vi "Rig - Save or Load.vi"(6 "Saving Rig Config to test directory?":bool, 7 "Rig Settings IN":T1={"Rig Name"="", "Rig Room"="1.4", "Base Directory"="", "Computer IP Address"="", "Globals Name"="", "Treatmill Str"="", "cRIO Test Data Dir"=path "", "ai"="", "ao"="", "dio"="", "A_calib_str_row1"="", "A_calib_str_row2"="0", "A_calib_str_row3"="1.4", "Zero_V_str"="", "step_V"="", "Sample Freq"="", "ai_threshold"="", "run_speed_thresh"="", "speed_time_length"="", "wall ball gain"="", "max wall pos"="", "max cor width"="", "Trial Config Directory"=path "C:/Whisker Tester/Trials", "Randomize Trials?"=FALSE}, 8 "Error IN":errorcluster, 10 "RigSave Path IN":path, 11 "Command IN":T2) -> (0 "Error OUT":errorcluster, 3 "Rig Settings OUT":T1={"Rig Name"="", "Rig Room"="1.4", "Base Directory"="", "Computer IP Address"="", "Globals Name"="", "Treatmill Str"="", "cRIO Test Data Dir"=path "", "ai"="", "ao"="", "dio"="", "A_calib_str_row1"="", "A_calib_str_row2"="0", "A_calib_str_row3"="1.4", "Zero_V_str"="", "step_V"="", "Sample Freq"="", "ai_threshold"="", "run_speed_thresh"="", "speed_time_length"="", "wall ball gain"="", "max wall pos"="", "max cor width"="", "Trial Config Directory"=path "C:/Whisker Tester/Trials", "Randomize Trials?"=FALSE})   [LabVIEW 2018]
uses:
  controls/Command IN_Recipe.ctl
  controls/Rig Config Settings.ctl
  <vilib>/Utility/file.llb/Write Delimited Spreadsheet (string).vi
  <vilib>/Utility/file.llb/Read Delimited Spreadsheet (string).vi
  Globals/Global - Configuration Options.vi
panel:
  # "INPUTS"
  # "OUTPUTS"
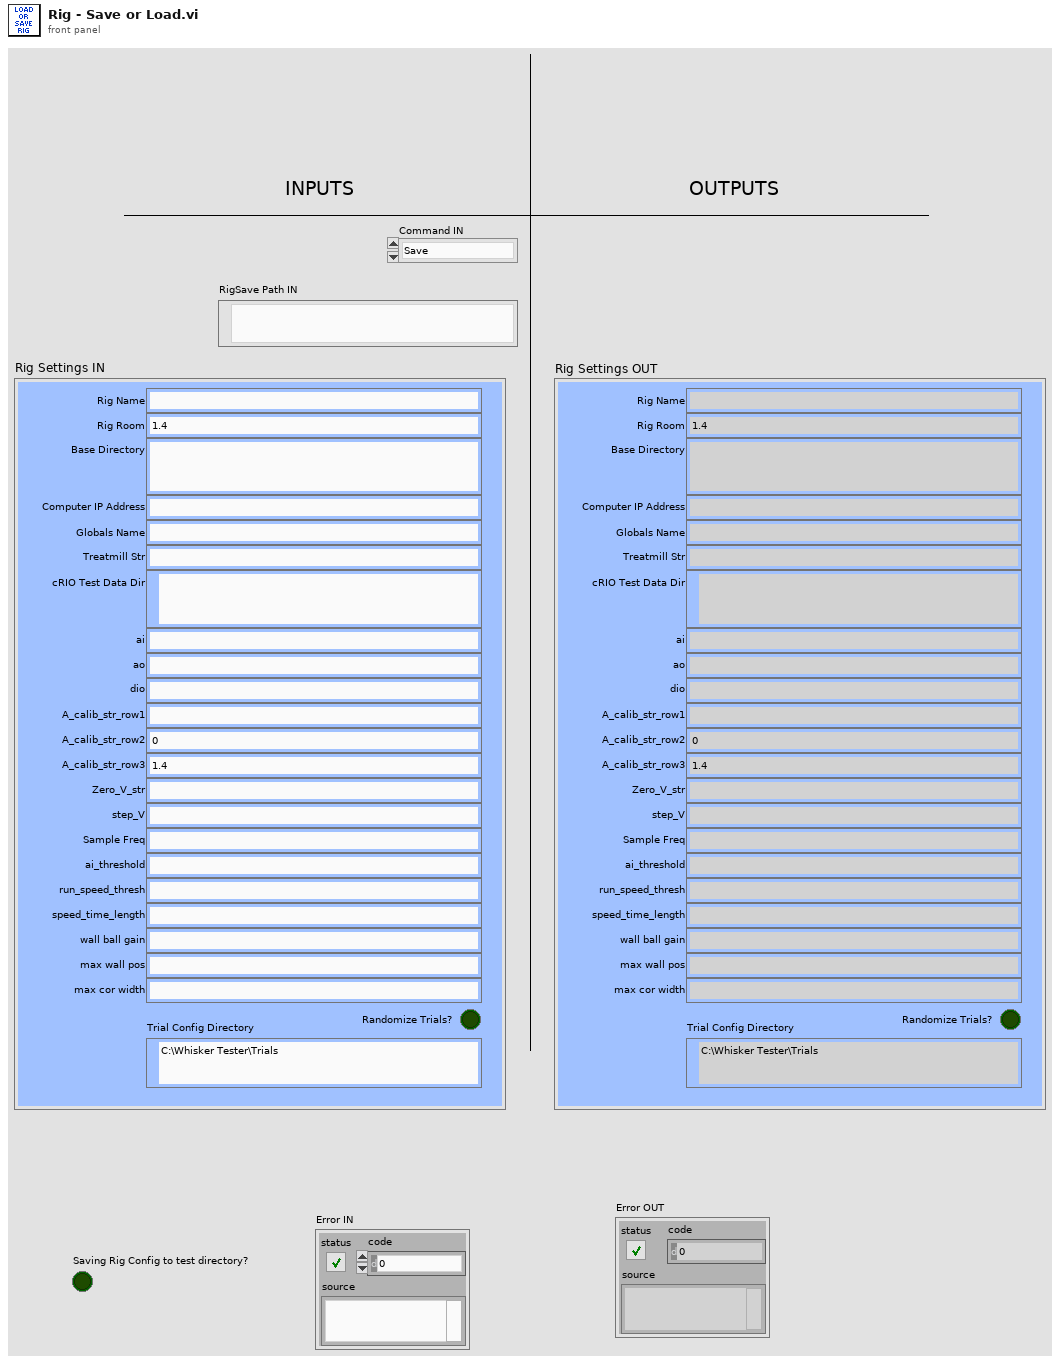
[diagram p1: front panel]
types:
  T1 = typedef "Rig Config Settings.ctl" = cluster{"Rig Name":string, "Rig Room":string, "Base Directory":string, "Computer IP Address":string, "Globals Name":string, "Treatmill Str":string, "cRIO Test Data Dir":path, "ai":string, "ao":string, "dio":string, "A_calib_str_row1":string, "A_calib_str_row2":string, "A_calib_str_row3":string, "Zero_V_str":string, "step_V":string, "Sample Freq":string, "ai_threshold":string, "run_speed_thresh":string, "speed_time_length":string, "wall ball gain":string, "max wall pos":string, "max cor width":string, "Trial Config Directory":path, "Randomize Trials?":bool}
  T2 = typedef "Command IN_Recipe.ctl" = enum16{"Save", "Load"}
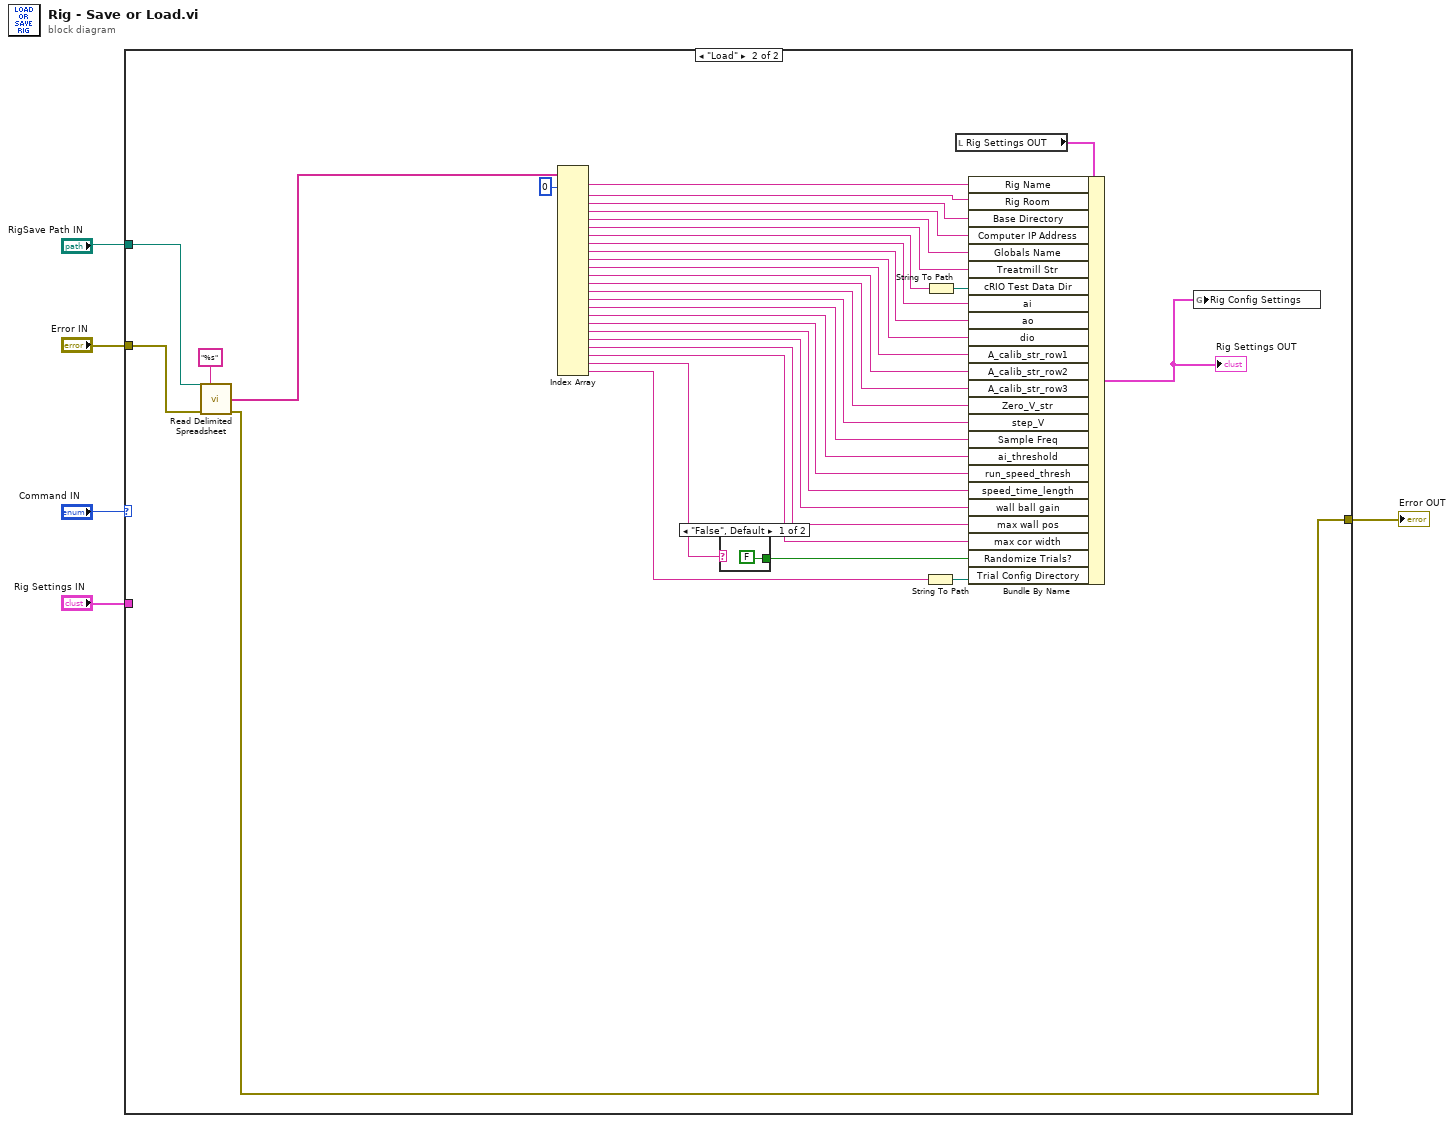
[diagram p0: block diagram]
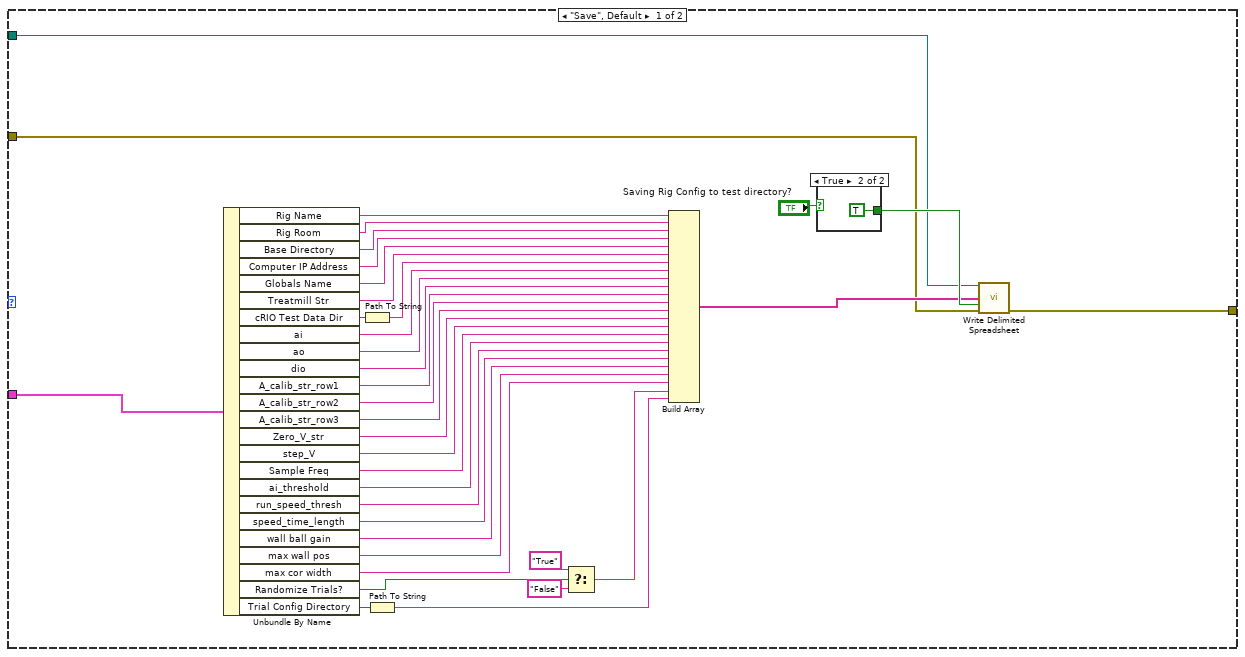
[diagram p2: hidden frame]
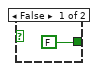
[diagram p3: hidden frame]
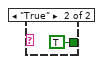
[diagram p4: hidden frame]
diagram:
  n1 = case shown="\"Load\"" "Command IN" {
    tunnel: "Rig Settings IN" -> [w35 _]
    tunnel: "RigSave Path IN" -> [w40 w77]
    tunnel: [w38 w75] -> w5
    tunnel: "Error IN" -> [w37 w76]
    frame "Save", Default {
      n2 = Unbundle By Name(w35) -> ("Rig Name"=w34:string, "Rig Room"=w33:string, "Base Directory"=w32:string, "Computer IP Address"=w31:string, "Globals Name"=w30:string, "Treatmill Str"=w29:string, "cRIO Test Data Dir"=w7:path, "ai"=w28:string, "ao"=w27:string, "dio"=w26:string, "A_calib_str_row1"=w25:string, "A_calib_str_row2"=w24:string, "A_calib_str_row3"=w23:string, "Zero_V_str"=w22:string, "step_V"=w21:string, "Sample Freq"=w20:string, "ai_threshold"=w19:string, "run_speed_thresh"=w18:string, "speed_time_length"=w17:string, "wall ball gain"=w16:string, "max wall pos"=w15:string, "max cor width"=w14:string, "Randomize Trials?"=w10:bool, "Trial Config Directory"=w13:path)
      n3 = Path To String(path=w7) -> (string=w6:string)
      n4 = Path To String(path=w13) -> (string=w8:string)
      n5 = Select(t="True", s=w10, f="False") -> (s? t:f=w9:string)
      n6 = Build Array(w34, w33, w32, w31, w30, w29, w6, w28, w27, w26, w25, w24, w23, w22, w21, w20, w19, w18, w17, w16, w15, w14, w9, w8) -> (w39:string[])
      n7 = case shown="True" "Saving Rig Config to test directory?" {
        tunnel: [FALSE ("append to file? (new file:F)") TRUE ("append to file? (new file:F)")] -> w41
        frame False {
        }
        frame True {
        }
      }
      n8 = call-poly <vilib>:"Write Delimited Spreadsheet.vi"("file path (dialog if empty)"=w40, "1D data"=w39, "append to file? (new file:F)"=w41, "error in (no error)"=w37) -> ("error out"=w38:errorcluster)  [unwired: 10 in, 1 out]
    }
    frame "Load" {
      n9 = call-poly <vilib>:"Read Delimited Spreadsheet.vi"("file path (dialog if empty)"=w77, "format (%s)"="%s" ("format (%.3f)"), "error in (no error)"=w76) -> ("first row"=w73:string[], "error out"=w75:errorcluster)  [unwired: 7 in, 4 out]
      n10 = Index Array(array=w73, index #1=0 ("index")) -> (element #1=w71:string, element #2=w70:string, element #3=w69:string, element #4=w68:string, element #5=w67:string, element #6=w66:string, element #7=w44:string, element #8=w65:string, element #9=w64:string, element #10=w63:string, element #11=w62:string, element #12=w61:string, element #13=w60:string, element #14=w59:string, element #15=w58:string, element #16=w57:string, element #17=w56:string, element #18=w55:string, element #19=w54:string, element #20=w53:string, element #21=w52:string, element #22=w51:string, element #23=w48:string, element #24=w46:string)  [unwired: 23 in]
      n11 = case shown="\"False\", Default" w48 {
        tunnel: [FALSE TRUE] -> w47
        frame "False", Default {
        }
        frame "True" {
        }
      }
      n12 = String To Path(string=w46) -> (path=w49:path)
      n13 = String To Path(string=w44) -> (path=w45:path)
      n14 = local read "Rig Settings OUT"() -> (w72:T1)
      n15 = Bundle By Name(cluster=w72, "Rig Name"=w71, "Rig Room"=w70, "Base Directory"=w69, "Computer IP Address"=w68, "Globals Name"=w67, "Treatmill Str"=w66, "cRIO Test Data Dir"=w45, "ai"=w65, "ao"=w64, "dio"=w63, "A_calib_str_row1"=w62, "A_calib_str_row2"=w61, "A_calib_str_row3"=w60, "Zero_V_str"=w59, "step_V"=w58, "Sample Freq"=w57, "ai_threshold"=w56, "run_speed_thresh"=w55, "speed_time_length"=w54, "wall ball gain"=w53, "max wall pos"=w52, "max cor width"=w51, "Randomize Trials?"=w47, "Trial Config Directory"=w49) -> (w50:T1)
      "Rig Settings OUT" <- w50
      n16 = global write "Global - Configuration Options.vi" "Rig Config Settings"(w50) -> ()
    }
  }
  "Error OUT" <- w5
